vi "Locate Devices.vi"(3 "error in (no error)":errorcluster) -> (0 "error out":errorcluster, 1 "Serial Numbers":string[](array[string]), 2 "Count":i32)   [LabVIEW 2017, in "OPA.OrpheusHP.lvclass"]
uses:
  OPA.OrpheusHP.lvclass
  E:/UPWORK/Laser Tool/Topas4PublicAPI/NET_SDK/Topas4Lib.dll
  Topas4PublicAPI/NET_SDK/Topas4Lib.dll
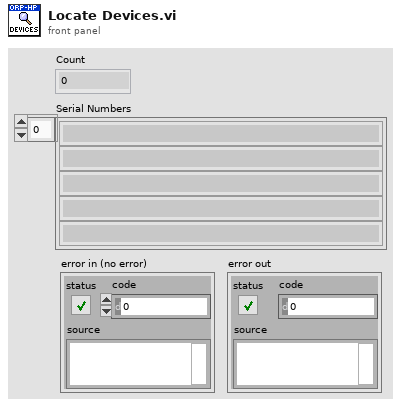
[diagram p1: front panel]
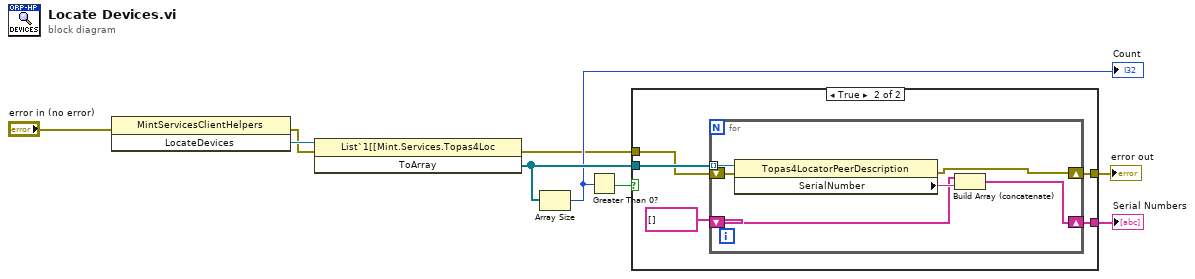
[diagram p0: block diagram]
diagram:
  n1 = invoke class="MintServicesClientHelpers" method="LocateDevices"(error in="error in (no error)") -> (error out=w3:errorcluster, "LocateDevices"=w9:refnum<k24>)  [unwired: 2 in, 1 out]
  n2 = invoke class="List`1[[Mint.Services.Topas4Loc" method="ToArray"(reference=w9, error in=w3) -> (error out=w2:errorcluster, "ToArray"=w8:refnum<k24>[])  [unwired: 1 in, 1 out]
  n3 = Array Size(array=w8) -> (size(s)=w7:i32)
  "Count" <- w7
  n4 = Greater Than 0?(x=w7) -> (x > 0?=w6:bool)
  n5 = case shown="True" w6 {
    tunnel: w8 -> [_ w15]
    tunnel: [_ w14] -> w5
    tunnel: w2 -> [w10 w12]
    tunnel: [w10 w11] -> w1
    frame False {
    }
    frame True {
      n6 = for {
        tunnel: w15 -> [w21] mode=indexing
        shift-right: [w19] -> w14
        shift-left: string[] [] ("appended array") -> [w18]
        shift-right: [w16] -> w11
        shift-left: w12 -> [w17]
        n7 = property class="Topas4LocatorPeerDescription"(reference=w21, error in=w17) -> (error out=w16:errorcluster, "SerialNumber"=w20:string)  [unwired: 1 out]
        n8 = Build Array (concatenate)(w18, w20) -> (w19:string[])
      }
    }
  }
  "Serial Numbers" <- w5
  "error out" <- w1
